vi "Camera Manager Get Current Version.vi"(8 "error in (no error)":errorcluster) -> (0 "error out":errorcluster, 3 "function return":string)   [LabVIEW 2017, in "PlayNitrideCameraComponet1010_4.lvlib"]
doc: "__declspec(dllexport) const char* CameraManager_GetCurrentVersion();"
uses:
  <userlib>/PlayNitrideCameraComponet1010_4/PlayNitrideCameraComponet1010_4.lvlib
  <userlib>/PlayNitrideCameraComponet1010_4/PlayNitrideCameraComponet.dll
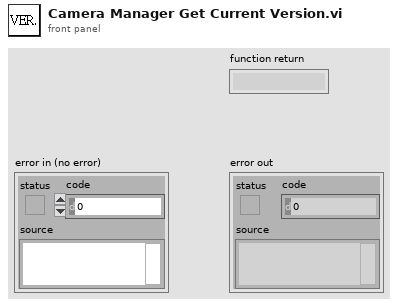
[diagram p1: front panel]
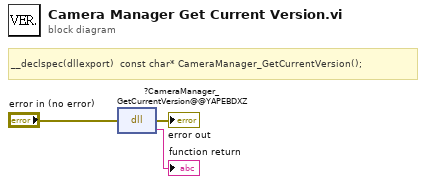
[diagram p0: block diagram]
diagram:
  # "__declspec(dllexport)  const char* CameraManager_GetCurrentVersion();"
  n1 = dll-call lib="C:/Program Files/National Instruments/LabVIEW 2017/user.lib/PlayNitrideCameraComponet1010_4/PlayNitrideCameraComponet.*" fn="?CameraManager_GetCurrentVersion@@YAPEBDXZ"(error in="error in (no error)") -> (error out=→"error out":errorcluster, →"function return":string)  [unwired: 2 in, 1 out]
